vi "fft.vi"() -> ()   [LabVIEW 2011]
uses:
  <vilib>/picture/cartesn2.llb/Waveform Plot Type.ctl
  <instrlib>/Tektronix DPO MSO 2000 4000 Series/Public/Data/Read (Single Waveform).vi
  <vilib>/express/express analysis/Spectral/Block/exnSpectralBlock spectral measurements RMS poly.vi
  <vilib>/express/express analysis/Spectral/Block/exnSpectralBlock spectral measurements RMS WFM.vi
  <vilib>/express/express analysis/Spectral/XNode/ExpressSpectralMeasurementsBlockNode.xnode
  <instrlib>/Tektronix DPO MSO 2000 4000 Series/Tektronix DPO MSO 2000 4000 Series.lvlib
panel:
  out "new picture":picture
  out "FFT - (RMS)":cluster{"f0":dbl, "df":dbl, "magnitude":dbl[]}
  out "Waveform Graph":waveform(dbl)(graph)
  in  "VISA resource name":refnum<visa-resource-name>
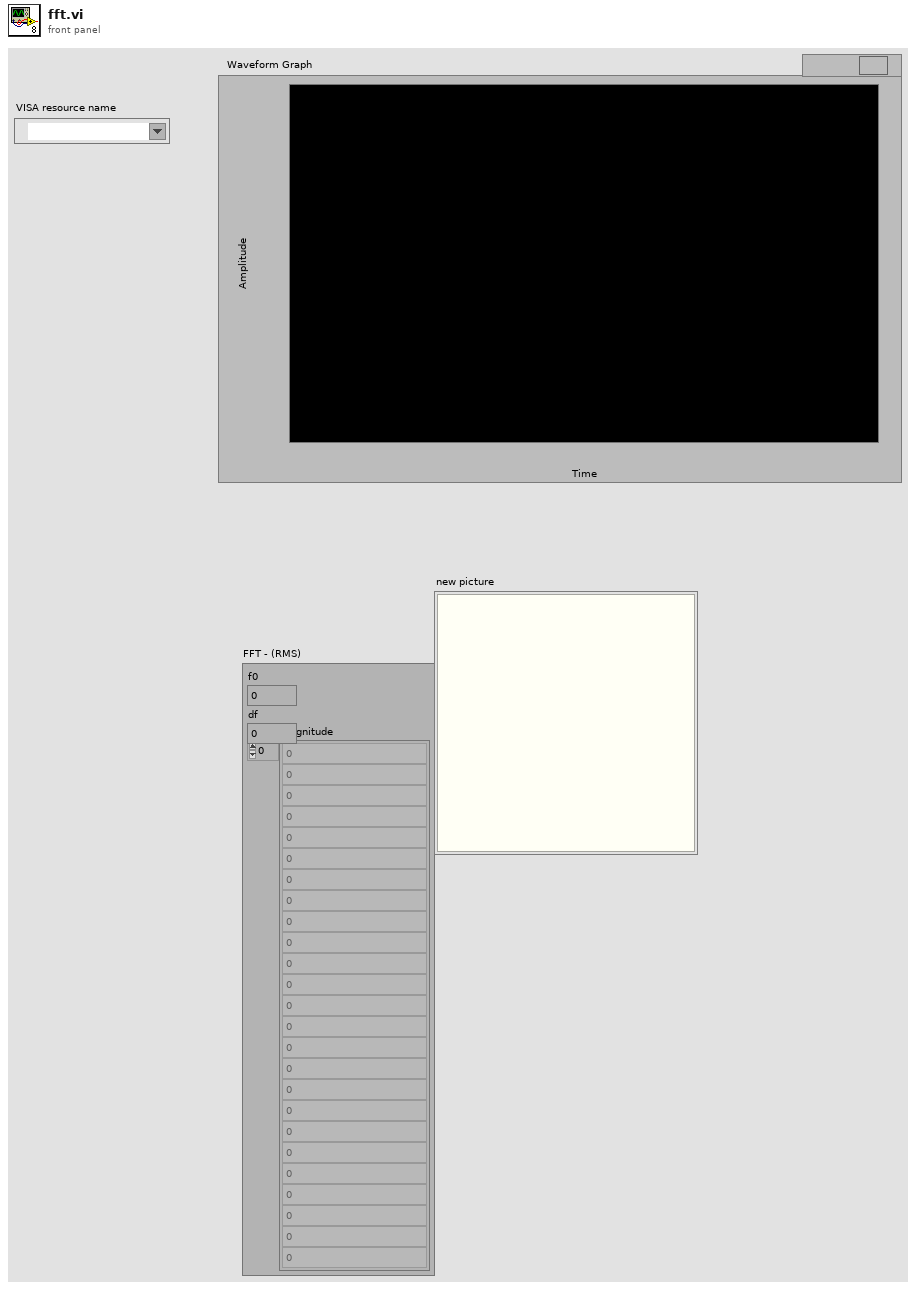
[diagram p1: front panel]
types:
  T1 = cluster{"bar width(50%)":dbl, "frame?(T)":bool, "frame color(black)":u32}
  T2 = cluster{"line color":u32, "text color":u32, "tick length(3)":i16, "crossing axes":bool, "visible grid?":bool}
  T3 = enum16{"User-specified Font", "Application Font", "System Font", "Dialog Font"}
  T4 = cluster{"Font Name:":string, "Size":i16, "Strikeout?":bool, "Italic?":bool, "Underline?":bool, "Outline?":bool, "Shadow?":bool, "Bold?":bool}
  T5 = cluster{"left":i16, "top":i16, "right":i16, "bottom":i16}
  T6 = cluster{"x minimum":dbl, "x maximum":dbl, "x log?":bool, "x precision":u8, "x format":enum8{"Decimal", "Scientific", "Engineering", "Binary", "Octal", "Hex"}, "y minimum":dbl, "y maximum":dbl, "y log?":bool, "y precision":u8, "y format":enum8{"Decimal", "Scientific", "Engineering", "Binary", "Octal", "Hex"}}
  T7 = typedef "Waveform Plot Type.ctl" = enum16{"points", "squares", "circles", "connected points", "connected squares", "connected circles", "fill to baseline", "comb plot", "bar plot"}
  T8 = cluster{"plot color":u32, "waveform plot type":T7, "baseline":dbl}
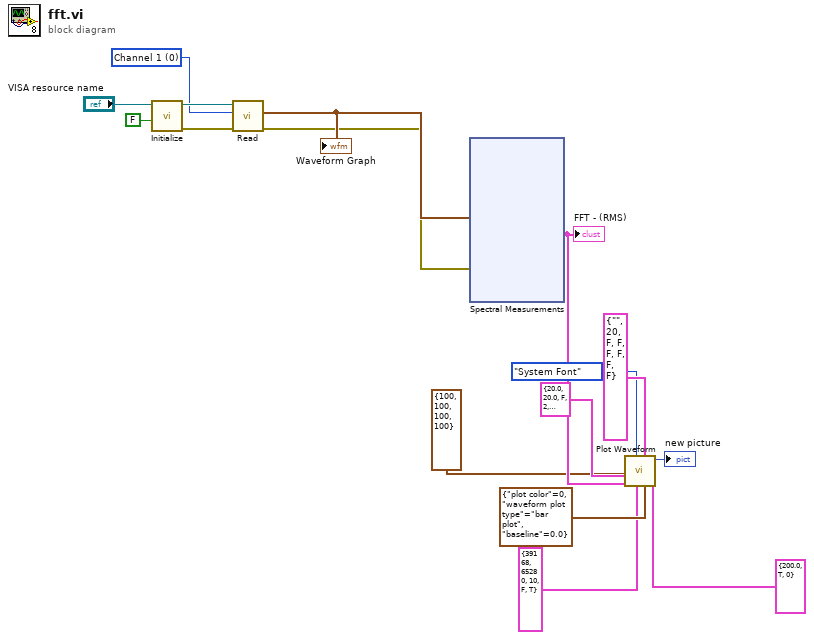
[diagram p0: block diagram]
diagram:
  w12 = u16 0 items=["Channel 1", "Channel 2", "Channel 3", "Channel 4", "Math", "Reference 1", "Reference 2", "Reference 3", "Reference 4", "D0", "D1", "D2", "D3", "D4", "D5", "D6", "D7", "D8", "D9", "D10", "D11", "D12", "D13", "D14", "D15", "Amplitude", "Frequency", "Phase", "Normal", "Average", "Maximum Peak Hold", "Minimum Peak Hold"] ("Channel (0: Channel 1)")
  n1 = call <instrlib>:"Initialize.vi"("Reset (True)"=FALSE, "VISA resource name"="VISA resource name") -> ("error out"=w14:errorcluster, "VISA resource name out"=w15:refnum<visa-resource-name>)  [unwired: 8 in]
  n2 = call-poly <instrlib>:"Read.vi"("error in (no error)"=w14, "Channel (0: Channel 1)"=w12, "VISA resource name"=w15) -> ("error out"=w10:errorcluster, "Waveform Graph"=w11:waveform(dbl))  [unwired: 6 in, 1 out]
  "Waveform Graph" <- w11
  n3 = xnode "Spectral Measurements"("Signals"=w11, "error in (no error)"=w10) -> ("FFT - (RMS)"=w9:cluster{"f0":dbl, "df":dbl, "magnitude":dbl[]})  [unwired: 2 out]
  "FFT - (RMS)" <- w9
  n4 = call <vilib>:"Plot Waveform.vi"("[bar style]"=T1 {"bar width(50%)"=200.0, "frame?(T)"=TRUE, "frame color(black)"=0}, "waveform plot cosmetics"=T8 {"plot color"=0, "waveform plot type"=enum."bar plot", "baseline"=0.0}, "[user-specified font]"=T4 {"Font Name:"="", "Size"=20, "Strikeout?"=FALSE, "Italic?"=FALSE, "Underline?"=FALSE, "Outline?"=FALSE, "Shadow?"=FALSE, "Bold?"=FALSE}, "cartesian grid cosmetics"=T2 {"line color"=39168, "text color"=65280, "tick length(3)"=10, "crossing axes"=FALSE, "visible grid?"=TRUE}, "desired font(Application)"=T3."System Font", "waveform data"=w9, "cartesian axis attributes"=T6 {"x minimum"=20.0, "x maximum"=20.0, "x log?"=FALSE, "x precision"=2, "x format"=enum."Decimal", "y minimum"=20.0, "y maximum"=20.0, "y log?"=FALSE, "y precision"=2, "y format"=enum."Decimal"}, "bounding rect"=T5 {"left"=100, "top"=100, "right"=100, "bottom"=100}) -> ("new picture"=→"new picture":picture)  [unwired: 3 in]
